vi "onTestExecution.vi"(7 "Name":string, 8 "error in (no error)":errorcluster, 11 "Test Runner.Project in":refnum<class "Test Runner.Class.lvclass">) -> (0 "error out":errorcluster, 3 "Test Runner.Project out":refnum<class "Test Runner.Class.lvclass">)   [LabVIEW 2013, in "Caraya.lvlib" / "Test Runner.Class.lvclass"]
uses:
  Test Runner.Class.lvclass
  Test Runner.Class.lvclass/Test Runner.Class.ctl
  Assert/Assert Not Error.vi
  Assert/Assert True.vi
  Assert/Assert.lvclass
  Test Runner/Test Runner.lvclass
  Test/Test.lvclass
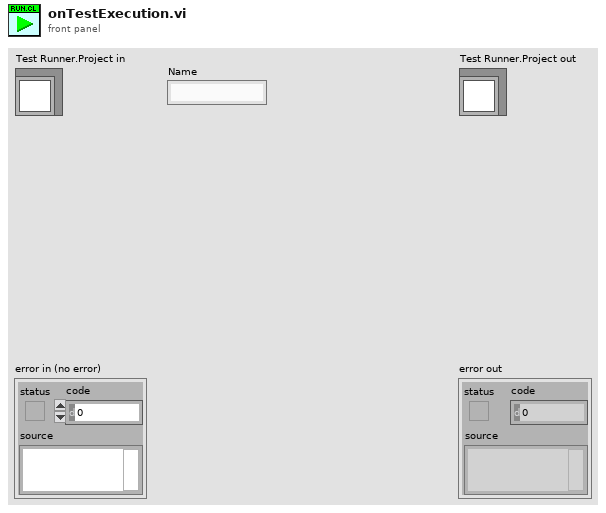
[diagram p1: front panel]
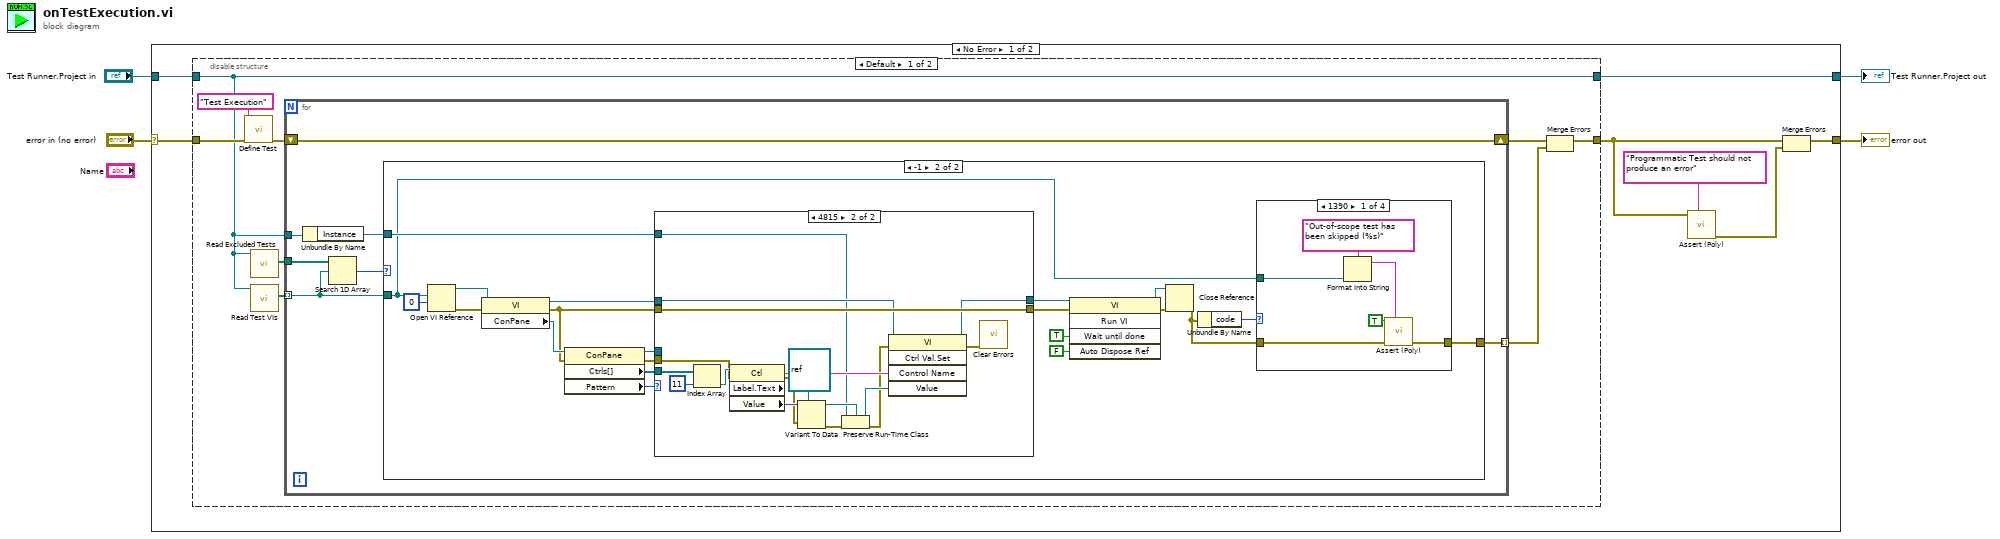
[diagram p0: block diagram]
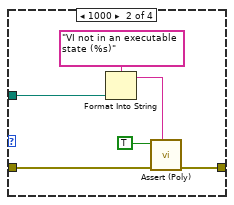
[diagram p4: hidden frame]
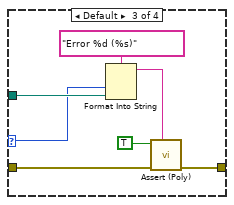
[diagram p5: hidden frame]
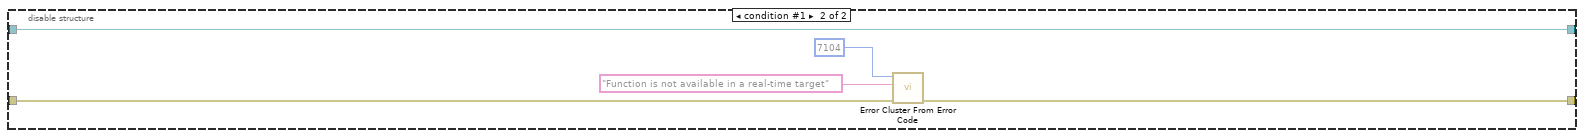
[diagram p7: hidden frame]
diagram:
  n1 = case shown="No Error" "error in (no error)" {
    selector: "error in (no error)" -> [w11 w94]
    tunnel: "Test Runner.Project in" -> [w6 w93]
    tunnel: [w5 w93] -> w4
    tunnel: [w10 w94] -> w3
    frame No Error {
      n2 = disable-structure shown="Default" {
        disable-tunnel: w11 -> [w17 w89]
        disable-tunnel: [w14 w88] -> w9
        disable-tunnel: w6 -> [w12 w92]
        disable-tunnel: [w12 w92] -> w5
        frame condition #0 (active) {
          n3 = call "Define Test.vi"("error in (no error)"=w17, "Label (VI Title)"="Test Execution") -> ("error out"=w16:errorcluster)  [unwired: 9 in]
          n4 = call "Read Excluded Tests.vi"("Test Runner in"=w12) -> ("Excluded Tests"=w19:path[])  [unwired: 8 in, 2 out]
          n5 = call "Read Test VIs.vi"("Test Runner in"=w12) -> ("Test VIs"=w18:path[])  [unwired: 8 in, 2 out]
          n6 = for {
            tunnel: w18 -> [w26] mode=indexing
            tunnel: [w25] -> w20 mode=indexing
            tunnel: w19 -> [w27]
            shift-right: [w23] -> w15
            shift-left: w16 -> [w23]
            tunnel: w12 -> [w22]
            n7 = Unbundle By Name(w22) -> ("Instance"=w21:refnum<class>)
            n8 = Search 1D Array(1D array=w27, element=w26) -> (index of element=w24:i32)  [unwired: 1 in]
            n9 = case shown="-1" w24 {
              tunnel: w26 -> [_ w29]
              tunnel: [_ w42] -> w25
              tunnel: w21 -> [_ w35]
              frame Default {
                # "Test is part of the exclusion list"
              }
              frame -1 {
                n10 = Open VI Reference(vi path=w29, options=0) -> (vi reference=w28:refnum<vi>, error out=w41:errorcluster)  [unwired: 4 in]
                n11 = property class="VI"(reference=w28, error in=w41) -> (reference out=w34:refnum<vi>, error out=w32:errorcluster, "ConPane"=w38:refnum<vi>)
                n12 = property class="ConPane"(reference=w38, error in=w32) -> (reference out=w37:refnum<vi>, error out=w36:errorcluster, "Ctrls[]"=w40:refnum<vi>[], "Pattern"=w39:u32)
                n13 = case shown="4815" w39 {
                  tunnel: w40 -> [_ w67]
                  tunnel: w37 -> [_ _]
                  tunnel: w36 -> [_ w61]
                  tunnel: w35 -> [_ w52]
                  tunnel: w34 -> [w50 w57]
                  tunnel: [w50 w56] -> w33
                  tunnel: w32 -> [w49 w59]
                  tunnel: [w49 w59] -> w31
                  frame 0, Default {
                  }
                  frame 4815 {
                    n14 = Index Array(array=w67, index=11) -> (element=w65:refnum<vi>)
                    n15 = property class="Ctl"(reference=w65, error in=w61) -> (error out=w60:errorcluster, "Label.Text"=w54:string, "Value"=w64:variant)  [unwired: 1 out]
                    n16 = Variant To Data(error in=w60, type=refnum<class> refnum ("Instance"), Variant=w64) -> (data=w53:refnum<class>, error out=w62:errorcluster)
                    n17 = Preserve Run-Time Class(object in=w52, error in=w62, 2:w53) -> (object out=w55:refnum<class>, error out=w51:errorcluster)
                    n18 = invoke on="Invoke Node" class="VI" method="Ctrl Val.Set"(reference=w57, error in=w51, "Control Name"=w54, "Value"=w55) -> (reference out=w56:refnum<vi>, error out=w58:errorcluster)  [unwired: 1 in, 3 out]
                    n19 = call <vilib>:"Clear Errors.vi"("error in (no error)"=w58) -> ()  [unwired: 6 in, 1 out]
                  }
                }
                n20 = invoke on="Invoke Node" class="VI" method="Run VI"(reference=w33, error in=w31, "Wait until done"=TRUE ("Wait Until Done"), "Auto Dispose Ref"=FALSE ("Auto Dispose Reference")) -> (reference out=w45:refnum<vi>, error out=w44:errorcluster)  [unwired: 1 in, 3 out]
                n21 = Close Reference(reference=w45, error in (no error)=w44) -> (error out=w43:errorcluster)
                n22 = Unbundle By Name(w43) -> ("code"=w46:i32)
                n23 = case shown="1390" w46 {
                  selector: w46 -> [_ _ w80 _]
                  tunnel: w43 -> [w72 w78 w85 w87]
                  tunnel: [w71 w77 w84 w87] -> w42
                  tunnel: w29 -> [w69 w75 w82 _]
                  frame 1390 {
                    n24 = Format Into String(format string="Out-of-scope test has been skipped (%s)" ("Label"), w69) -> (resulting string=w70:string)  [unwired: 2 in, 1 out]
                    n25 = call-poly "Assert (Poly).vi"("Label"=w70, "error in (no error)"=w72, "True?"=TRUE) -> ("error out"=w71:errorcluster)  [unwired: 8 in]
                  }
                  frame 1000 {
                    n26 = Format Into String(format string="VI not in an executable state (%s)" ("Label"), w75) -> (resulting string=w76:string)  [unwired: 2 in, 1 out]
                    n27 = call-poly "Assert (Poly).vi"("Label"=w76, "error in (no error)"=w78, "True?"=TRUE) -> ("error out"=w77:errorcluster)  [unwired: 8 in]
                  }
                  frame Default {
                    n28 = Format Into String(format string="Error %d (%s)" ("Label"), w80, w82) -> (resulting string=w83:string)  [unwired: 2 in, 1 out]
                    n29 = call-poly "Assert (Poly).vi"("Label"=w83, "error in (no error)"=w85, "True?"=TRUE) -> ("error out"=w84:errorcluster)  [unwired: 8 in]
                  }
                  frame 0 {
                  }
                }
              }
            }
          }
          n30 = Merge Errors(w15, w20) -> (w14:errorcluster)
        }
        frame condition #1 {
          n31 = call <vilib>:"Error Cluster From Error Code.vi"("error in (no error)"=w89, "error message (\"\")"="Function is not available in a real-time target" ("error message (\"\")"), "error code (0)"=7104) -> ("error out"=w88:errorcluster)  [unwired: 6 in]
        }
      }
      n32 = call-poly "Assert (Poly).vi"("Label"="Programmatic Test should not produce an error", "Not Error?"=w9) -> ("error out"=w7:errorcluster)  [unwired: 9 in]
      n33 = Merge Errors(w9, w7) -> (w10:errorcluster)
    }
    frame Error {
    }
  }
  "error out" <- w3
  "Test Runner.Project out" <- w4
